vi "Farming Robot V3.vi"() -> ()   [LabVIEW 2021]
uses:
  <vilib>/myRIO/Express VI/Onboard Devices/LED/LED Express VI.xnode
  <vilib>/myRIO/Instrument Drivers/Onboard IO/DIO/vis/Write.vi
  <vilib>/myRIO/Instrument Drivers/Onboard IO/DIO/DIO.lvlib
  <vilib>/myRIO/Common/Instrument Driver Framework/myRIO v1.0/DIO/typedefs/DIO Channels Enum.ctl
  <vilib>/myRIO/Common/Instrument Driver Framework/myRIO v1.0/DIO/typedefs/DIO Channels List.ctl
  <vilib>/myRIO/Common/Instrument Driver Framework/Utilities/typedefs/Generic FPGA Reference.ctl
  <vilib>/myRIO/Common/Instrument Driver Framework/Utilities/typedefs/myRIO v1.0 Reference.ctl
  <vilib>/myRIO/Common/Instrument Driver Framework/Utilities/typedefs/Hardware Version Enum.ctl
  <vilib>/myRIO/Common/Instrument Driver Framework/Utilities/typedefs/myRIO Generic Hardware Reference.ctl
  <vilib>/myRIO/Instrument Drivers/Onboard IO/DIO/typedefs/DIO Reference.ctl
  <vilib>/myRIO/Instrument Drivers/Onboard IO/DIO/vis/myRIO DIO Open.xnode
  <vilib>/myRIO/Common/Instrument Driver Framework/Utilities/vis/Is FPGA Ref Available.vi
  <vilib>/myRIO/Common/Instrument Driver Framework/myRIO v1.0/DIO/vis/myRIO v1.1 Open DIO.vi
  <vilib>/userDefined/High Color/nirio_resource_hc.ctl
  <vilib>/myRIO/Express VI/Onboard IO/DO/DO Express VI.xnode
  <vilib>/myRIO/Instrument Drivers/Onboard IO/PWM/typedefs/PWM Configuration.ctl
  <vilib>/myRIO/Instrument Drivers/Onboard IO/PWM/PWM.lvlib
  <vilib>/myRIO/Common/Instrument Driver Framework/myRIO v1.0/PWM/typedefs/PWM Channels Enum.ctl
  <vilib>/myRIO/Instrument Drivers/Onboard IO/PWM/typedefs/PWM Reference.ctl
  <vilib>/myRIO/Instrument Drivers/Onboard IO/PWM/vis/Set Duty Cycle and Frequency.vi
  <vilib>/myRIO/Common/Instrument Driver Framework/myRIO v1.0/PWM/vis/myRIO v1.1 Open PWM.vi
  <vilib>/myRIO/Instrument Drivers/Onboard IO/PWM/vis/myRIO PWM Open.xnode
  <vilib>/myRIO/Express VI/Onboard IO/PWM/PWM Express VI.xnode
  <vilib>/myRIO/Common/Instrument Driver Framework/myRIO v1.0/Accelerometer/typedefs/Accelerometer Channels Enum.ctl
  <vilib>/myRIO/Common/Instrument Driver Framework/myRIO v1.0/Accelerometer/typedefs/Accelerometer Channels List.ctl
  <vilib>/myRIO/Instrument Drivers/Onboard Devices/Accelerometer/typedefs/Accelerometer Reference.ctl
  <vilib>/myRIO/Instrument Drivers/Onboard Devices/Accelerometer/Accelerometer.lvlib
  <vilib>/myRIO/Instrument Drivers/Onboard Devices/Accelerometer/vis/Read.vi
  <vilib>/myRIO/Common/Instrument Driver Framework/myRIO v1.0/Accelerometer/vis/myRIO v1.1 Open Accelerometer.vi
  <vilib>/myRIO/Instrument Drivers/Onboard Devices/Accelerometer/vis/myRIO Accelerometer Open.xnode
  <vilib>/myRIO/Express VI/Onboard Devices/Accelerometer/Accelerometer Express VI.xnode
panel:
  in  "Start Farming":bool
  out "Enum":T1(ring)
  out "pulse width 2":dbl
  out "Angle 2":dbl
  out "pulse width 1":dbl
  out "Angle 1":dbl
  out "Watering":bool
  out "Seeding\nUp":bool
  out "Seeding\nDown":bool
  out "Switching\nMode":bool
  out "Drill Up":bool
  out "Drill Down":bool
  out "Intialize":bool
  out "Message":string
  in  "stop":bool
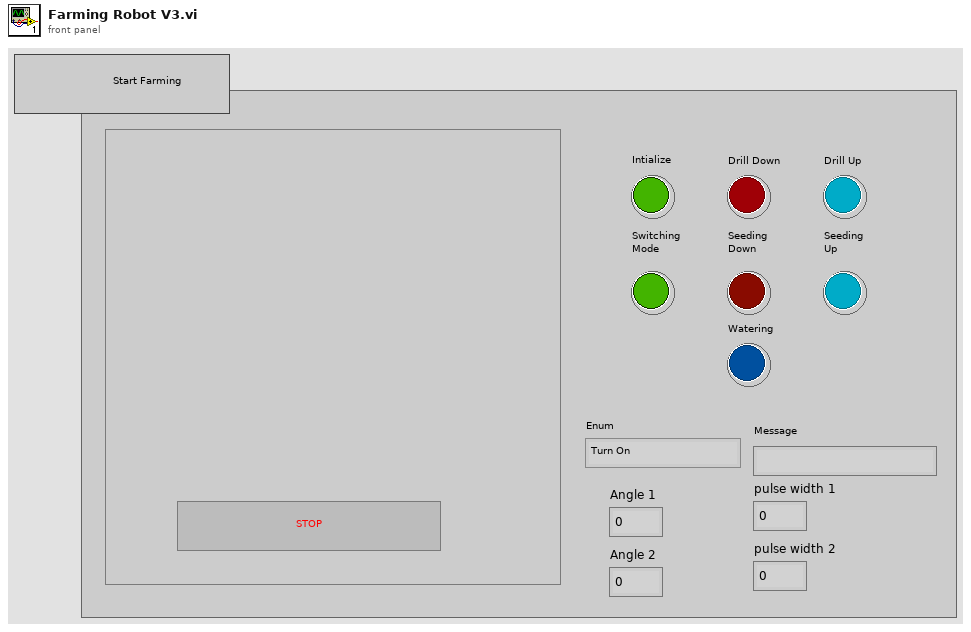
[diagram p1: front panel]
types:
  T1 = enum16{"Turn On", "IDLE", "Start farming", "Drive", "Drilling", "Seeding", "Watering", "Filling", "Fell Off", "Stop"}
  T2 = typedef "DIO.lvlib/DIO Reference.ctl" = cluster{"myRIO Reference":T3, "DIO Channels List":T7}
  T3 = typedef "myRIO Generic Hardware Reference.ctl" = cluster{"myRIO Model":T4, "myRIO Hardware Reference":T5}
  T4 = typedef "Hardware Version Enum.ctl" = enum16{"Unknown", "myRIO-1900", "myRIO-1950", "roboRIO", "NI ELVIS RIO CM", "ELVIS III"}
  T5 = typedef "myRIO v1.0 Reference.ctl" = cluster{"Generic FPGA Reference":T6, "Allow multiple opens":bool}
  T6 = typedef "Generic FPGA Reference.ctl" = refnum<k20>
  T7 = typedef "DIO Channels List.ctl" = T8[]
  T8 = typedef "DIO Channels Enum.ctl" = enum16{"Not Connected", "C/DIO0", "C/DIO1", "C/DIO2", "C/DIO3", "C/DIO4", "C/DIO5", "C/DIO6", "C/DIO7", "A/DIO0", "A/DIO1", "A/DIO2", "A/DIO3", "A/DIO4", "A/DIO5", "A/DIO6", "A/DIO7", "A/DIO8", "A/DIO9", "A/DIO10", "A/DIO11", "A/DIO12", "A/DIO13", "A/DIO14", "A/DIO15", "A/DIO16", "A/DIO17", "A/DIO18", "A/DIO19", "B/DIO0", "B/DIO1", "B/DIO2", "B/DIO3", "B/DIO4", "B/DIO5", "B/DIO6", "B/DIO7", "B/DIO8", "B/DIO9", "B/DIO10", "B/DIO11", "B/DIO12", "B/DIO13", "B/DIO14", "B/DIO15", "B/DIO16", "B/DIO17", "B/DIO18", "B/DIO19", "LED0", "LED1", "LED2", "LED3", "Button0", "DIO/DIO0", "DIO/DIO1", "DIO/DIO2", "DIO/DIO3", "DIO/DIO4", "DIO/DIO5", "DIO/DIO6", "DIO/DIO7", "DIO/DIO8", "DIO/DIO9", "SPI/CS0", "SPI/CS1", "SPI/CS2", "SPI/CS3", "LED RADIO (Green)", "LED RADIO (Red)", "LED COMM (Green)", "LED COMM (Red)", "LED MODE (Green)", "LED MODE (Red)"}
  T9 = typedef "nirio_resource_hc.ctl" = tag
  T10 = typedef "Accelerometer.lvlib/Accelerometer Reference.ctl" = cluster{"myRIO Reference":T3, "Accelerometer Channels List":T11, "LSB Weight":dbl}
  T11 = typedef "Accelerometer Channels List.ctl" = T12[]
  T12 = typedef "Accelerometer Channels Enum.ctl" = enum16{"Not Connected", "X-Axis", "Y-Axis", "Z-Axis"}
  T13 = typedef "PWM.lvlib/PWM Reference.ctl" = cluster{"myRIO Reference":T3, "PWM Channels Enum":T14, "PWM Configuration":T15}
  T14 = typedef "PWM Channels Enum.ctl" = enum16{"Not Connected", "C/PWM0", "C/PWM1", "A/PWM0", "A/PWM1", "A/PWM2", "A/PWM3", "A/PWM4", "A/PWM5", "A/PWM6", "A/PWM7", "A/PWM8", "A/PWM9", "A/PWM10", "A/PWM11", "A/PWM12", "A/PWM13", "A/PWM14", "A/PWM15", "A/PWM16", "A/PWM17", "A/PWM18", "A/PWM19", "B/PWM0", "B/PWM1", "B/PWM2", "B/PWM3", "B/PWM4", "B/PWM5", "B/PWM6", "B/PWM7", "B/PWM8", "B/PWM9", "B/PWM10", "B/PWM11", "B/PWM12", "B/PWM13", "B/PWM14", "B/PWM15", "B/PWM16", "B/PWM17", "B/PWM18", "B/PWM19", "PWM/PWM0", "PWM/PWM1", "PWM/PWM2", "PWM/PWM3", "PWM/PWM4", "PWM/PWM5", "PWM/PWM6", "PWM/PWM7", "PWM/PWM8", "PWM/PWM9"}
  T15 = typedef "PWM.lvlib/PWM Configuration.ctl" = cluster{"Frequency":dbl, "Duty Cycle":dbl}
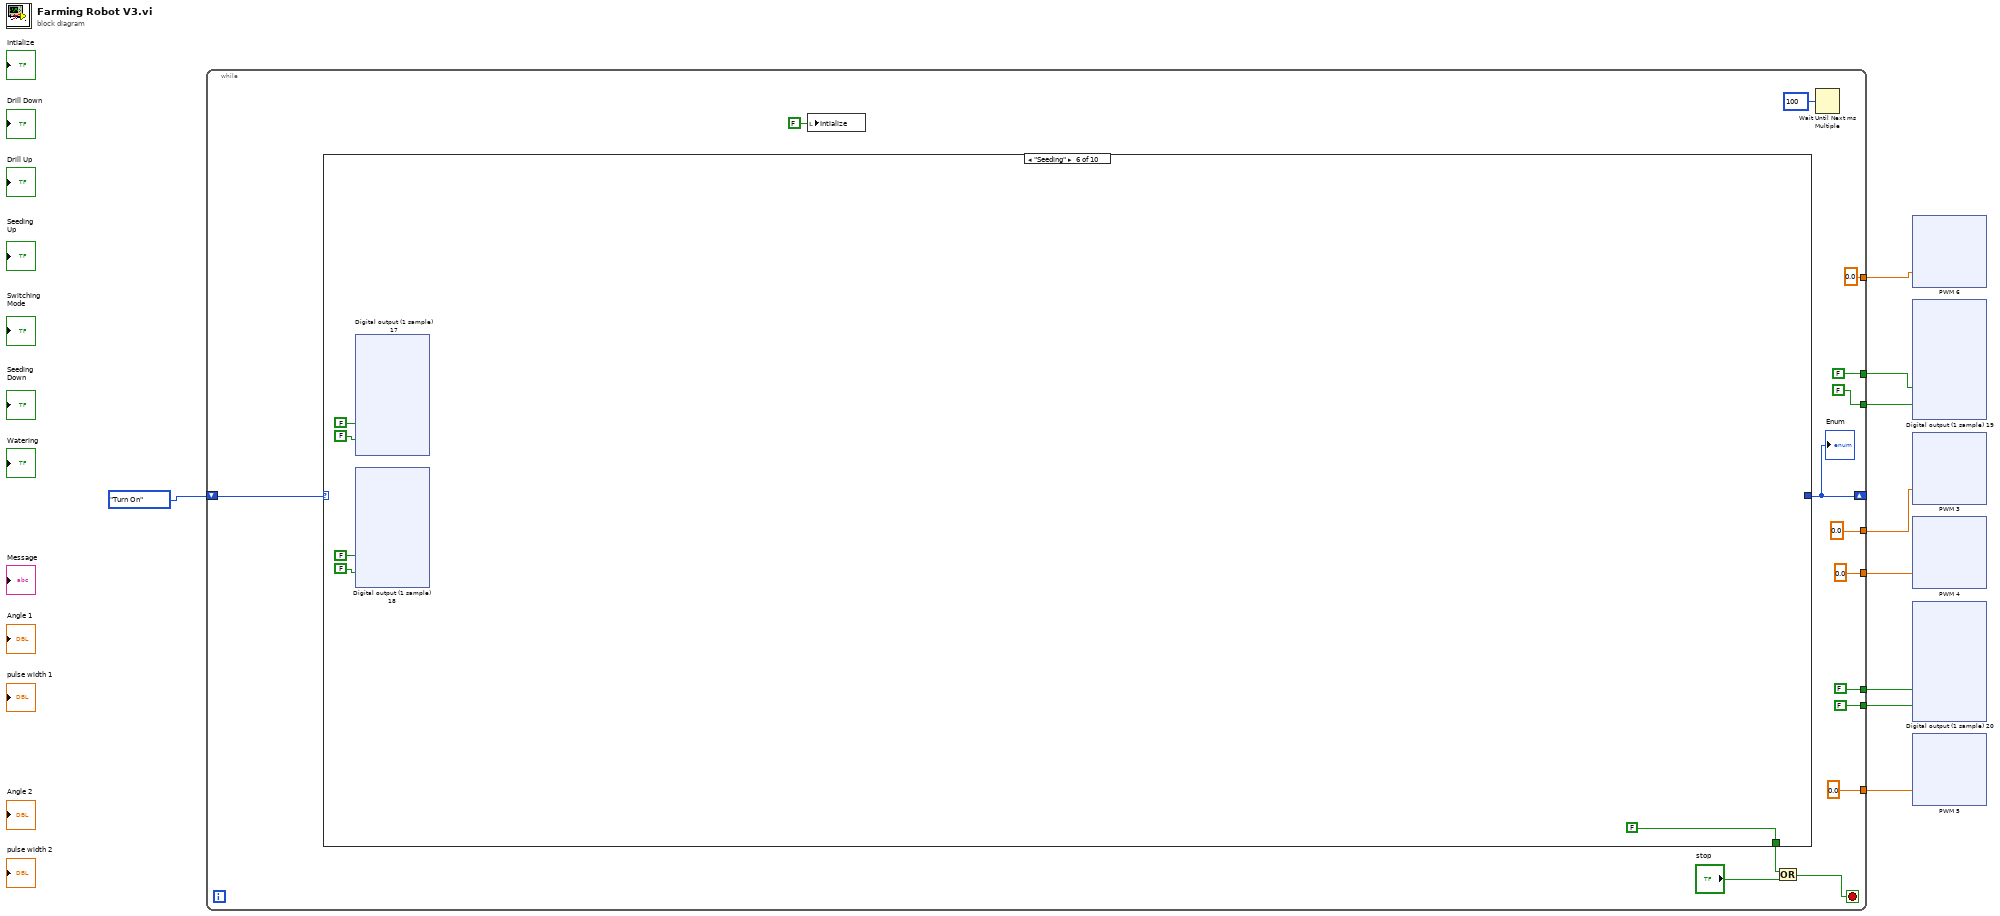
[diagram p0: block diagram]
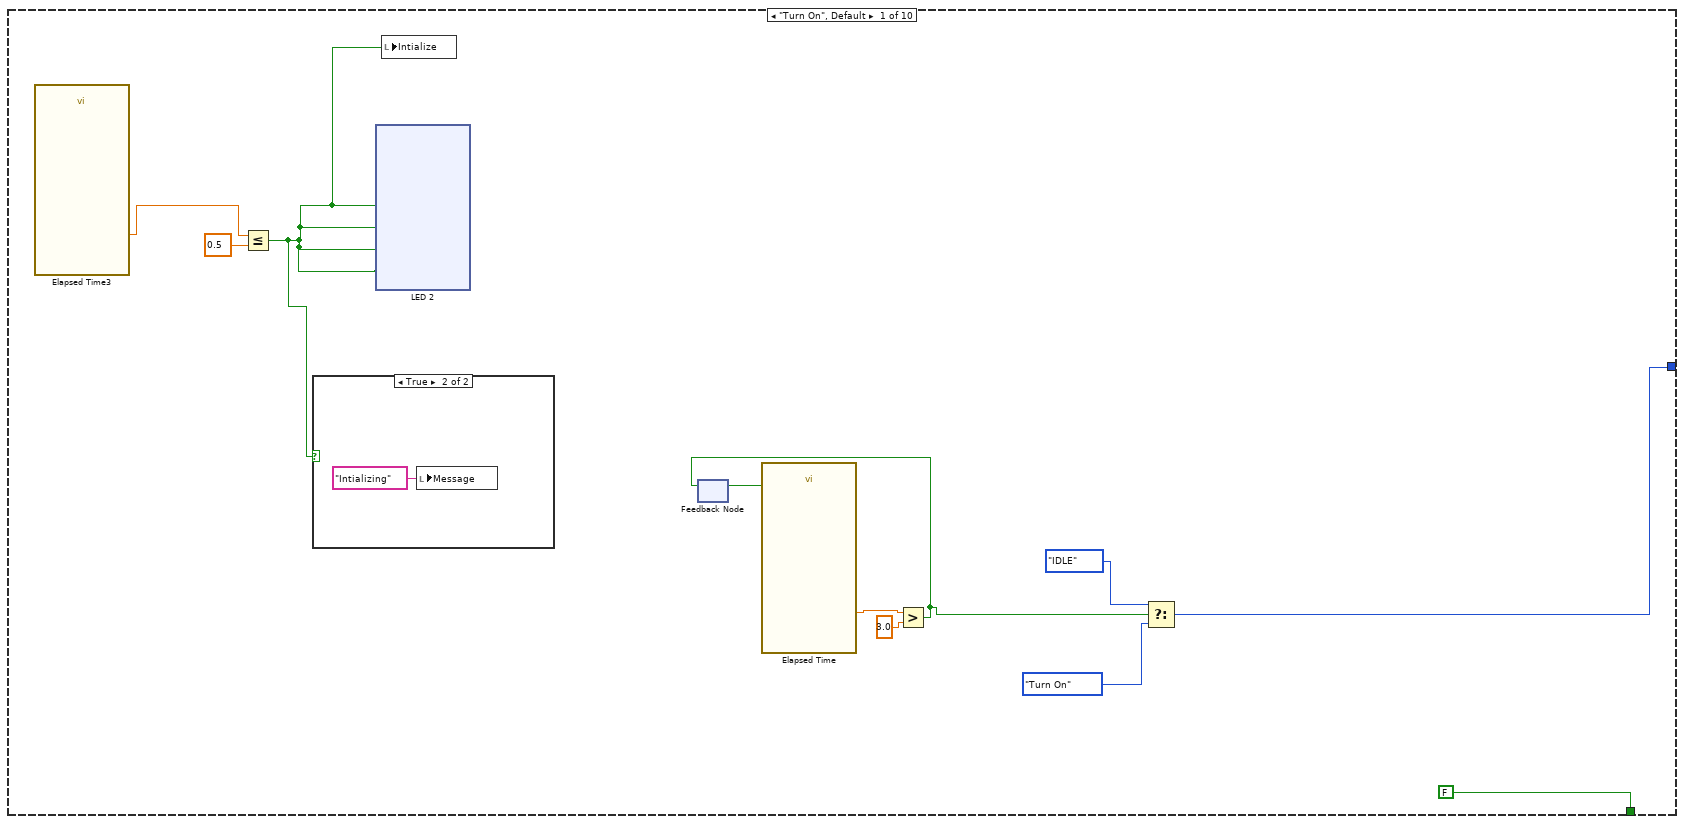
[diagram p2: hidden frame]
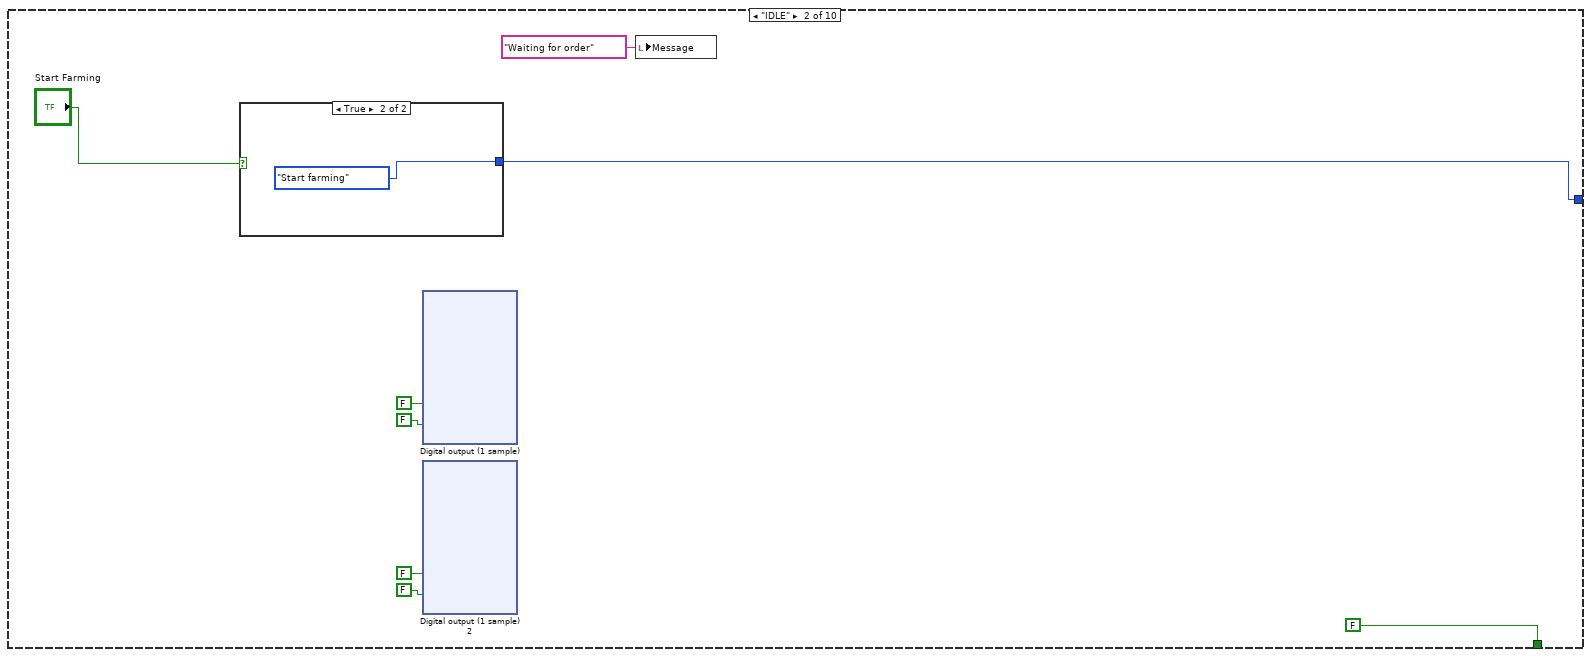
[diagram p4: hidden frame]
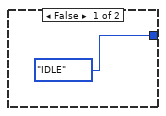
[diagram p5: hidden frame]
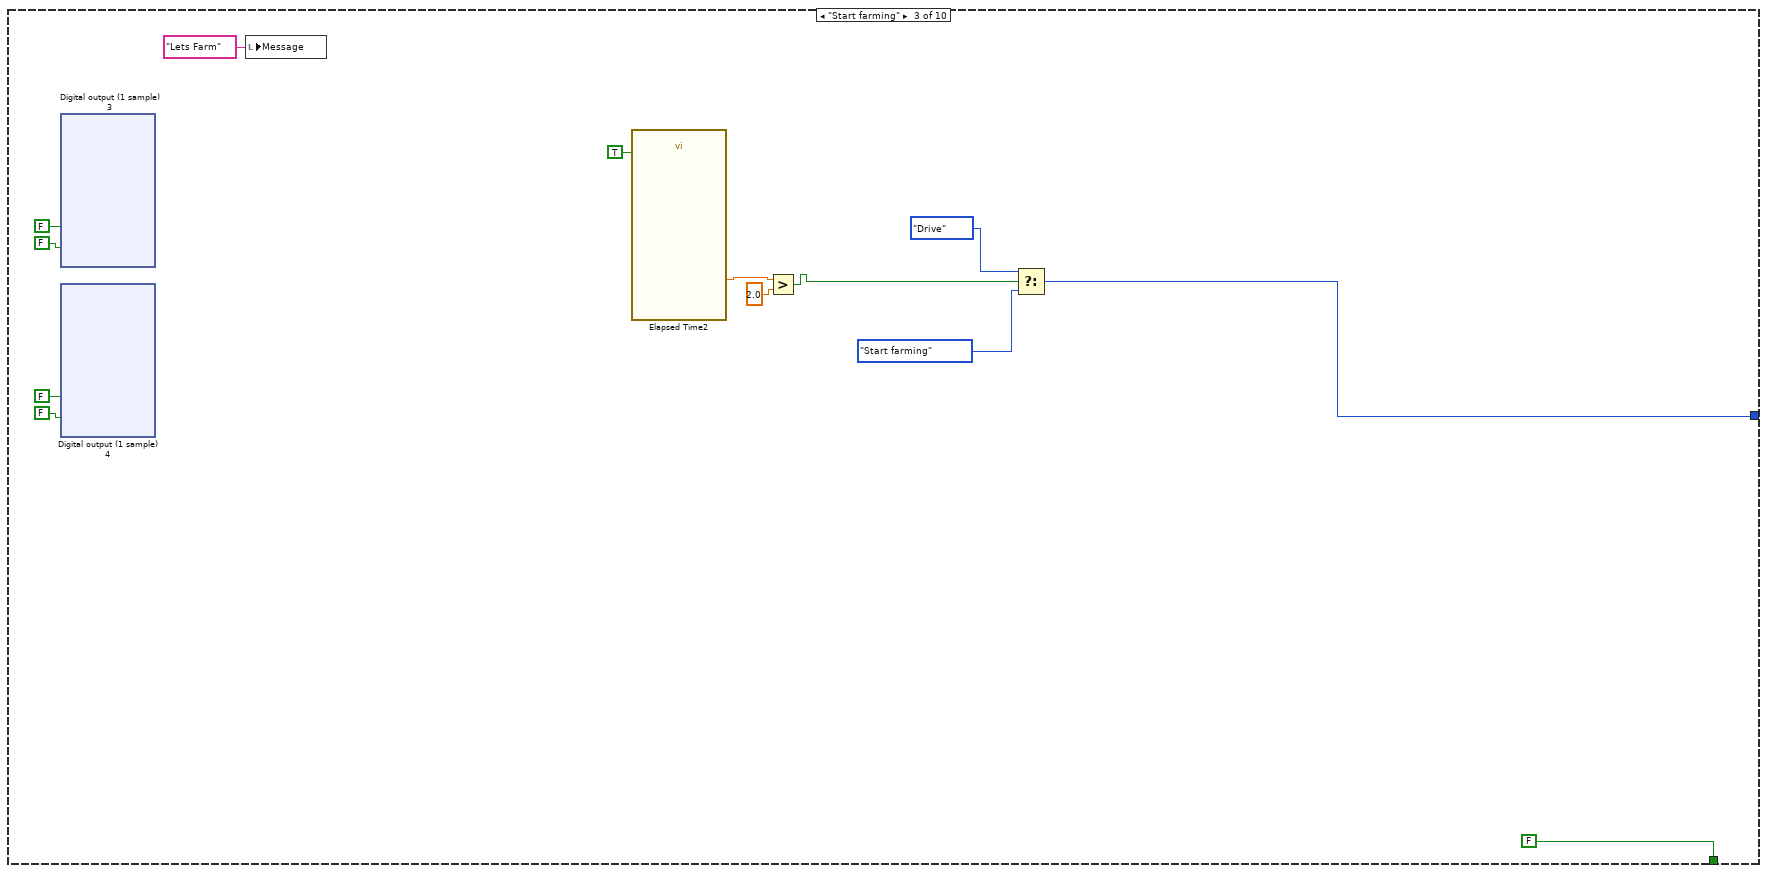
[diagram p6: hidden frame]
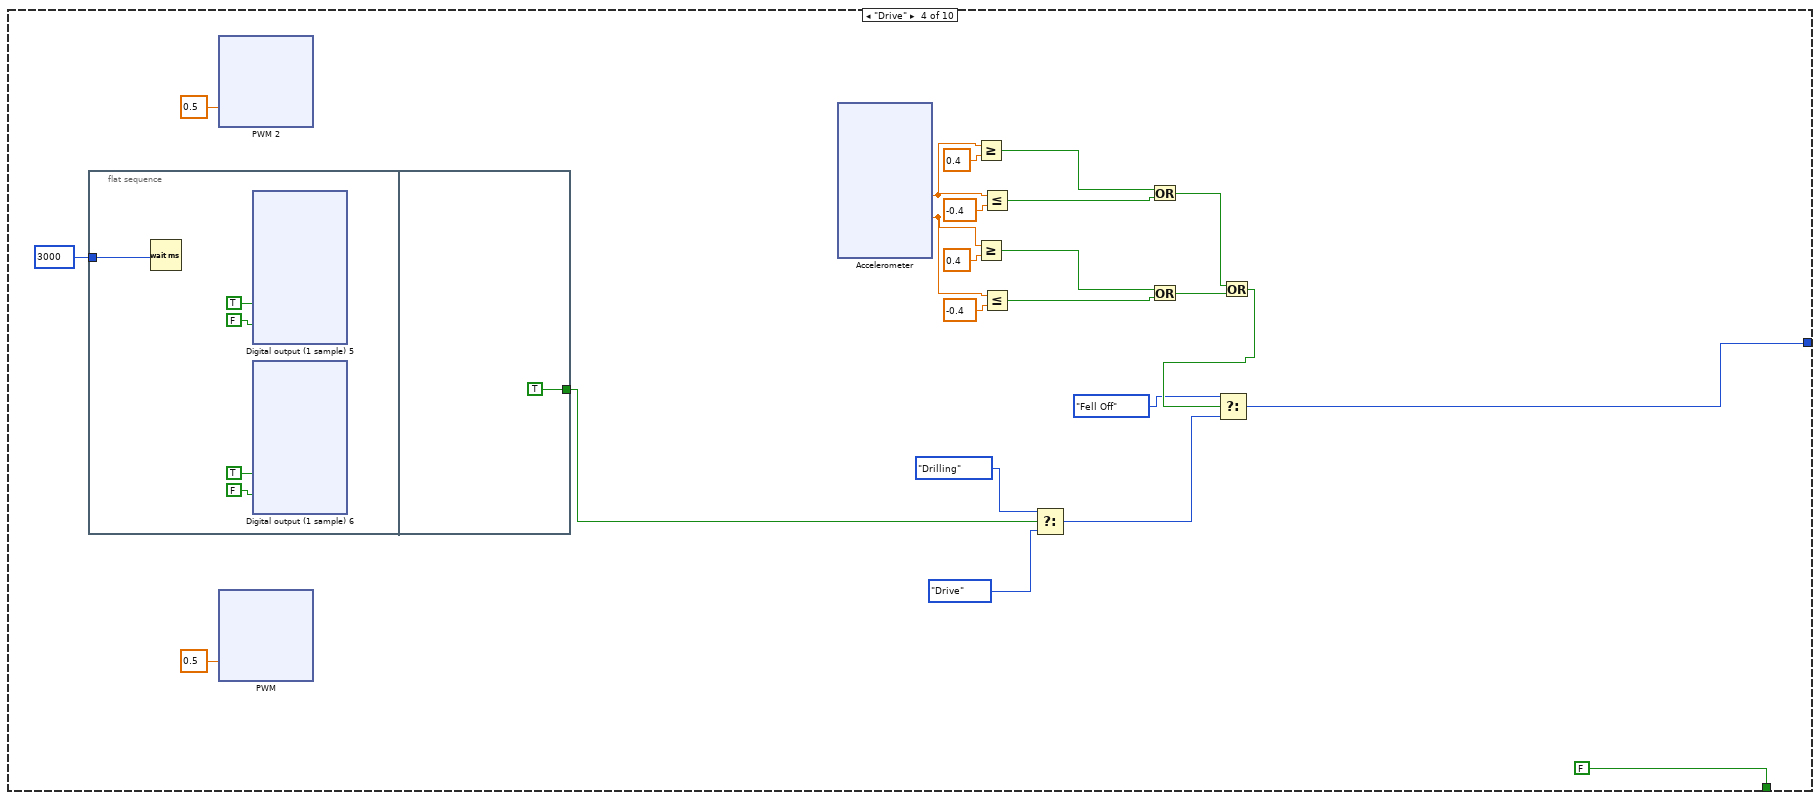
[diagram p7: hidden frame]
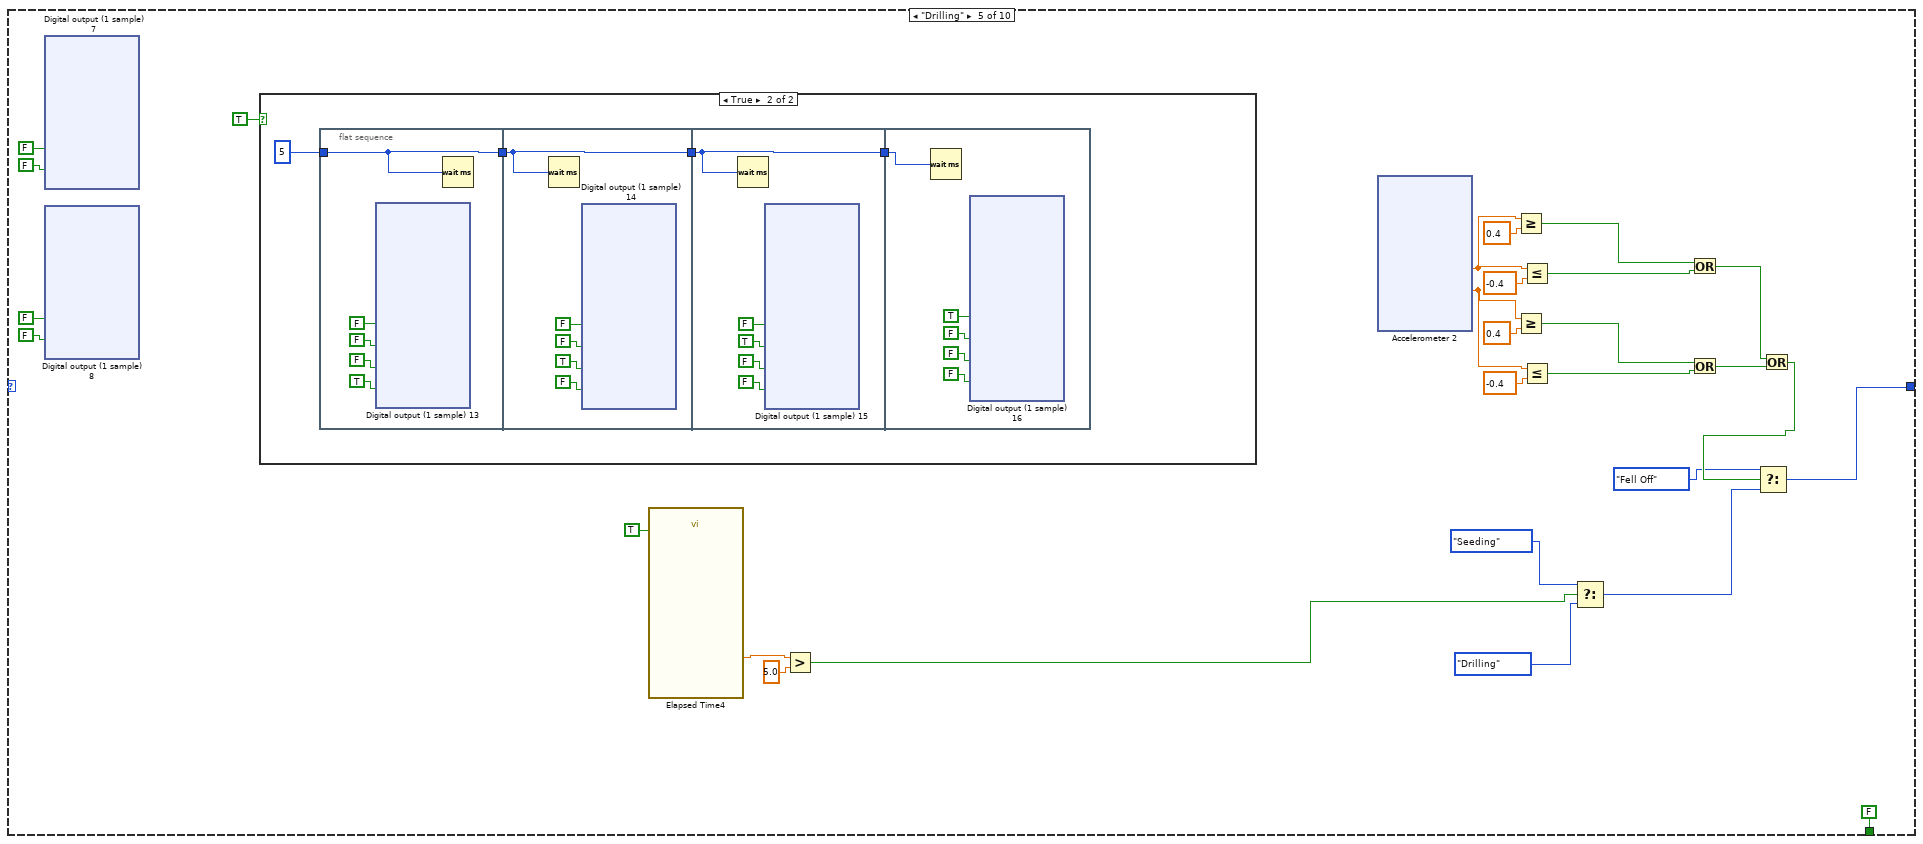
[diagram p8: hidden frame]
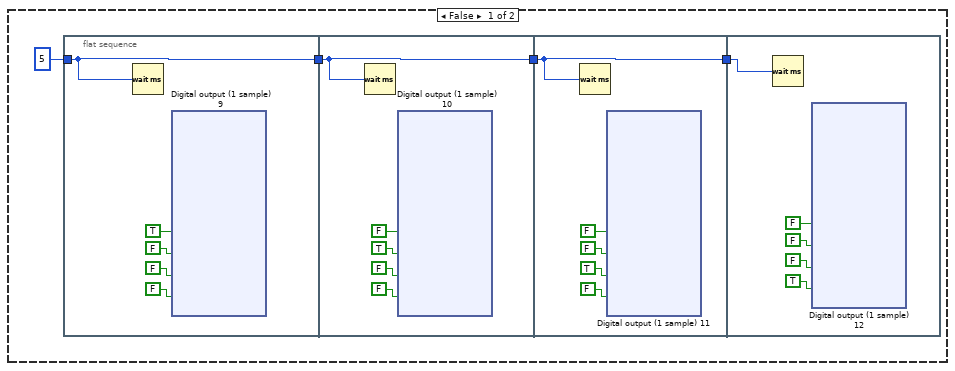
[diagram p9: hidden frame]
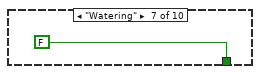
[diagram p10: hidden frame]
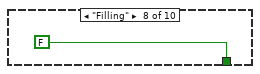
[diagram p11: hidden frame]
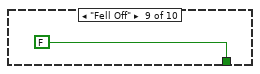
[diagram p12: hidden frame]
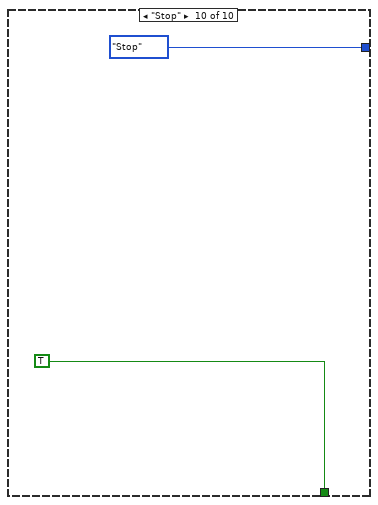
[diagram p13: hidden frame]
diagram:
  n1 = while {
    shift-right: [w20] -> _
    shift-left: T1."Turn On" ("Enum") -> [w22]
    tunnel: [0.0 ("Duty Cycle")] -> w8
    tunnel: [FALSE ("A/DIO1 (Pin 13)")] -> w7
    tunnel: [FALSE ("A/DIO0 (Pin 11)")] -> w6
    tunnel: [0.0 ("Duty Cycle")] -> w5
    tunnel: [0.0 ("Duty Cycle")] -> w4
    tunnel: [FALSE ("A/DIO3 (Pin 17)")] -> w3
    tunnel: [FALSE ("A/DIO2 (Pin 15)")] -> w2
    tunnel: [0.0 ("Duty Cycle")] -> w1
    stop <- w24 stop-if-true
    n2 = case shown="\"Seeding\"" w22 {
      tunnel: [w26 w81 w159 w245 w452 _ _ _ _ T1."Stop" ("Enum")] -> w20
      tunnel: [FALSE ("x") FALSE ("x") FALSE ("x") FALSE ("x") FALSE ("x") FALSE ("x") FALSE ("x") FALSE ("x") FALSE ("x") TRUE ("x")] -> w18
      frame "Turn On", Default {
        n3 = call "Elapsed Time3"() -> ("Elapsed Time (s)"=w34:dbl)  [unwired: 12 in, 7 out]
        n4 = Less Or Equal?(x=w34, y=0.5) -> (x <= y?=w33:bool)
        n5 = case shown="True" w33 {
          frame False {
          }
          frame True {
            n6 = local write "Message"("Intializing" ("Message")) -> ()
          }
        }
        n7 = xnode "LED 2"("LED0"=w33, "LED1"=w33, "LED2"=w33, "LED3"=w33) -> ()  [unwired: 1 in, 1 out]
        n8 = local write "Intialize"(w33) -> ()
        n9 = feedback #1() -> (w30:bool)  [unwired: 1 in]
        n10 = call "Elapsed Time"("Reset"=w30) -> ("Elapsed Time (s)"=w32:dbl)  [unwired: 11 in, 7 out]
        n11 = Greater?(x=w32, y=3.0) -> (0:w27:bool)
        n12 = feedback-in #1(w27) -> ()
        n13 = Select(t=T1."IDLE" ("Enum"), s=w27, f=T1."Turn On" ("Enum")) -> (s? t:f=w26:T1)
      }
      frame "IDLE" {
        n14 = case shown="True" "Start Farming" {
          tunnel: [T1."IDLE" ("Enum") T1."Start farming" ("Enum")] -> w81
          frame False {
          }
          frame True {
          }
        }
        n15 = xnode "Digital output (1 sample)"("A/DIO0 (Pin 11)"=FALSE, "A/DIO1 (Pin 13)"=FALSE) -> ()  [unwired: 1 in, 1 out]
        n16 = xnode "Digital output (1 sample) 2"("A/DIO2 (Pin 15)"=FALSE, "A/DIO3 (Pin 17)"=FALSE) -> ()  [unwired: 1 in, 1 out]
        n17 = local write "Message"("Waiting for order" ("Message")) -> ()
      }
      frame "Start farming" {
        n18 = xnode "Digital output (1 sample) 3"("A/DIO0 (Pin 11)"=FALSE, "A/DIO1 (Pin 13)"=FALSE) -> ()  [unwired: 1 in, 1 out]
        n19 = xnode "Digital output (1 sample) 4"("A/DIO2 (Pin 15)"=FALSE, "A/DIO3 (Pin 17)"=FALSE) -> ()  [unwired: 1 in, 1 out]
        n20 = local write "Message"("Lets Farm" ("Message")) -> ()
        n21 = call "Elapsed Time2"("Reset"=TRUE) -> ("Elapsed Time (s)"=w164:dbl)  [unwired: 11 in, 7 out]
        n22 = Greater?(x=w164, y=2.0) -> (0:w160:bool)
        n23 = Select(t=T1."Drive" ("Enum"), s=w160, f=T1."Start farming" ("Enum")) -> (s? t:f=w159:T1)
      }
      frame "Drive" {
        n24 = flat-sequence {
          tunnel: u32 3000 ("milliseconds to wait") -> [w304]
          tunnel: [TRUE ("s")] -> w247
          frame #0 {
            n25 = Wait (ms)(milliseconds to wait=w304) -> ()  [unwired: 1 out]
            n26 = xnode "Digital output (1 sample) 5"("A/DIO2 (Pin 15)"=TRUE, "A/DIO3 (Pin 17)"=FALSE) -> ()  [unwired: 1 in, 1 out]
            n27 = xnode "Digital output (1 sample) 6"("A/DIO0 (Pin 11)"=TRUE, "A/DIO1 (Pin 13)"=FALSE) -> ()  [unwired: 1 in, 1 out]
          }
          frame #1 {
          }
        }
        n28 = xnode "PWM 2"("Duty Cycle"=0.5) -> ()  [unwired: 1 in, 1 out]
        n29 = xnode "PWM"("Duty Cycle"=0.5) -> ()  [unwired: 1 in, 1 out]
        n30 = xnode "Accelerometer"() -> ("X-Axis"=w262:dbl, "Y-Axis"=w251:dbl)  [unwired: 1 in, 2 out]
        n31 = Greater Or Equal?(x=w262, y=0.4) -> (x >= y?=w259:bool)
        n32 = Greater Or Equal?(x=w251, y=0.4) -> (x >= y?=w253:bool)
        n33 = Less Or Equal?(x=w262, y=-0.4) -> (x <= y?=w258:bool)
        n34 = Less Or Equal?(x=w251, y=-0.4) -> (x <= y?=w252:bool)
        n35 = Select(t=T1."Drilling" ("Enum"), s=w247, f=T1."Drive" ("Enum")) -> (s? t:f=w244:T1)
        n36 = Or(x=w259, y=w258) -> (x .or. y?=w257:bool)
        n37 = Or(x=w253, y=w252) -> (x .or. y?=w256:bool)
        n38 = Or(x=w257, y=w256) -> (x .or. y?=w246:bool)
        n39 = Select(t=T1."Fell Off" ("Enum"), s=w246, f=w244) -> (s? t:f=w245:T1)
      }
      frame "Drilling" {
        n40 = xnode "Digital output (1 sample) 7"("A/DIO0 (Pin 11)"=FALSE, "A/DIO1 (Pin 13)"=FALSE) -> ()  [unwired: 1 in, 1 out]
        n41 = xnode "Digital output (1 sample) 8"("A/DIO2 (Pin 15)"=FALSE, "A/DIO3 (Pin 17)"=FALSE) -> ()  [unwired: 1 in, 1 out]
        n42 = case shown="True" TRUE {
          frame False {
            n43 = flat-sequence {
              tunnel: u32 5 ("milliseconds to wait") -> [w527]
              tunnel: [w527] -> w522
              tunnel: [w570] -> w521
              tunnel: w522 -> [w570]
              tunnel: [w613] -> w520
              tunnel: w521 -> [w613]
              tunnel: w520 -> [w656]
              frame #0 {
                n44 = Wait (ms)(milliseconds to wait=w527) -> ()  [unwired: 1 out]
                n45 = xnode "Digital output (1 sample) 9"("B/DIO0 (Pin 11)"=TRUE, "B/DIO1 (Pin 13)"=FALSE, "B/DIO2 (Pin 15)"=FALSE, "B/DIO3 (Pin 17)"=FALSE) -> ()  [unwired: 1 in, 1 out]
              }
              frame #1 {
                n46 = Wait (ms)(milliseconds to wait=w570) -> ()  [unwired: 1 out]
                n47 = xnode "Digital output (1 sample) 10"("B/DIO0 (Pin 11)"=FALSE, "B/DIO1 (Pin 13)"=TRUE, "B/DIO2 (Pin 15)"=FALSE, "B/DIO3 (Pin 17)"=FALSE) -> ()  [unwired: 1 in, 1 out]
              }
              frame #2 {
                n48 = Wait (ms)(milliseconds to wait=w613) -> ()  [unwired: 1 out]
                n49 = xnode "Digital output (1 sample) 11"("B/DIO0 (Pin 11)"=FALSE, "B/DIO1 (Pin 13)"=FALSE, "B/DIO2 (Pin 15)"=TRUE, "B/DIO3 (Pin 17)"=FALSE) -> ()  [unwired: 1 in, 1 out]
              }
              frame #3 {
                n50 = Wait (ms)(milliseconds to wait=w656) -> ()  [unwired: 1 out]
                n51 = xnode "Digital output (1 sample) 12"("B/DIO0 (Pin 11)"=FALSE, "B/DIO1 (Pin 13)"=FALSE, "B/DIO2 (Pin 15)"=FALSE, "B/DIO3 (Pin 17)"=TRUE) -> ()  [unwired: 1 in, 1 out]
              }
            }
          }
          frame True {
            n52 = flat-sequence {
              tunnel: u32 5 ("milliseconds to wait") -> [w703]
              tunnel: [w703] -> w695
              tunnel: [w746] -> w696
              tunnel: w695 -> [w746]
              tunnel: [w789] -> w697
              tunnel: w696 -> [w789]
              tunnel: w697 -> [w832]
              frame #0 {
                n53 = xnode "Digital output (1 sample) 13"("B/DIO0 (Pin 11)"=FALSE, "B/DIO1 (Pin 13)"=FALSE, "B/DIO2 (Pin 15)"=FALSE, "B/DIO3 (Pin 17)"=TRUE) -> ()  [unwired: 1 in, 1 out]
                n54 = Wait (ms)(milliseconds to wait=w703) -> ()  [unwired: 1 out]
              }
              frame #1 {
                n55 = Wait (ms)(milliseconds to wait=w746) -> ()  [unwired: 1 out]
                n56 = xnode "Digital output (1 sample) 14"("B/DIO0 (Pin 11)"=FALSE, "B/DIO1 (Pin 13)"=FALSE, "B/DIO2 (Pin 15)"=TRUE, "B/DIO3 (Pin 17)"=FALSE) -> ()  [unwired: 1 in, 1 out]
              }
              frame #2 {
                n57 = Wait (ms)(milliseconds to wait=w789) -> ()  [unwired: 1 out]
                n58 = xnode "Digital output (1 sample) 15"("B/DIO0 (Pin 11)"=FALSE, "B/DIO1 (Pin 13)"=TRUE, "B/DIO2 (Pin 15)"=FALSE, "B/DIO3 (Pin 17)"=FALSE) -> ()  [unwired: 1 in, 1 out]
              }
              frame #3 {
                n59 = Wait (ms)(milliseconds to wait=w832) -> ()  [unwired: 1 out]
                n60 = xnode "Digital output (1 sample) 16"("B/DIO0 (Pin 11)"=TRUE, "B/DIO1 (Pin 13)"=FALSE, "B/DIO2 (Pin 15)"=FALSE, "B/DIO3 (Pin 17)"=FALSE) -> ()  [unwired: 1 in, 1 out]
              }
            }
          }
        }
        n61 = call "Elapsed Time4"("Reset"=TRUE) -> ("Elapsed Time (s)"=w456:dbl)  [unwired: 11 in, 7 out]
        n62 = Greater?(x=w456, y=5.0) -> (0:w453:bool)
        n63 = xnode "Accelerometer 2"() -> ("X-Axis"=w473:dbl, "Y-Axis"=w462:dbl)  [unwired: 1 in, 2 out]
        n64 = Greater Or Equal?(x=w473, y=0.4) -> (x >= y?=w470:bool)
        n65 = Greater Or Equal?(x=w462, y=0.4) -> (x >= y?=w464:bool)
        n66 = Less Or Equal?(x=w473, y=-0.4) -> (x <= y?=w469:bool)
        n67 = Less Or Equal?(x=w462, y=-0.4) -> (x <= y?=w463:bool)
        n68 = Select(t=T1."Seeding" ("Enum"), s=w453, f=T1."Drilling" ("Enum")) -> (s? t:f=w458:T1)
        n69 = Or(x=w470, y=w469) -> (x .or. y?=w468:bool)
        n70 = Or(x=w464, y=w463) -> (x .or. y?=w467:bool)
        n71 = Or(x=w468, y=w467) -> (x .or. y?=w459:bool)
        n72 = Select(t=T1."Fell Off" ("Enum"), s=w459, f=w458) -> (s? t:f=w452:T1)
      }
      frame "Seeding" {
        n73 = xnode "Digital output (1 sample) 17"("A/DIO0 (Pin 11)"=FALSE, "A/DIO1 (Pin 13)"=FALSE) -> ()  [unwired: 1 in, 1 out]
        n74 = xnode "Digital output (1 sample) 18"("A/DIO2 (Pin 15)"=FALSE, "A/DIO3 (Pin 17)"=FALSE) -> ()  [unwired: 1 in, 1 out]
      }
      frame "Watering" {
      }
      frame "Filling" {
      }
      frame "Fell Off" {
      }
      frame "Stop" {
      }
    }
    "Enum" <- w20
    n75 = local write "Intialize"(FALSE ("Intialize")) -> ()
    n76 = Or(x=w18, y="stop") -> (x .or. y?=w24:bool)
    n77 = Wait Until Next ms Multiple(millisecond multiple=u32 100) -> ()  [unwired: 1 out]
  }
  n78 = xnode "PWM 6"("Duty Cycle"=w8) -> ()  [unwired: 1 in, 1 out]
  n79 = xnode "Digital output (1 sample) 19"("A/DIO0 (Pin 11)"=w6, "A/DIO1 (Pin 13)"=w7) -> ()  [unwired: 1 in, 1 out]
  n80 = xnode "PWM 3"("Duty Cycle"=w5) -> ()  [unwired: 1 in, 1 out]
  n81 = xnode "PWM 4"("Duty Cycle"=w4) -> ()  [unwired: 1 in, 1 out]
  n82 = xnode "Digital output (1 sample) 20"("A/DIO2 (Pin 15)"=w2, "A/DIO3 (Pin 17)"=w3) -> ()  [unwired: 1 in, 1 out]
  n83 = xnode "PWM 5"("Duty Cycle"=w1) -> ()  [unwired: 1 in, 1 out]
